vi "C8855_read_data.vi"(6 "error in (no error)":errorcluster, 7 "Cluster in":T1, 8 "Handle":i32) -> (0 "error out":errorcluster, 1 "Data update error 1":bool, 2 "Result Returned":u8, 3 "Handle 2":i32, 5 "Cluster out":T1)   [LabVIEW 2014]
uses:
  Source Cluster.ctl
  C8855-01api.dll
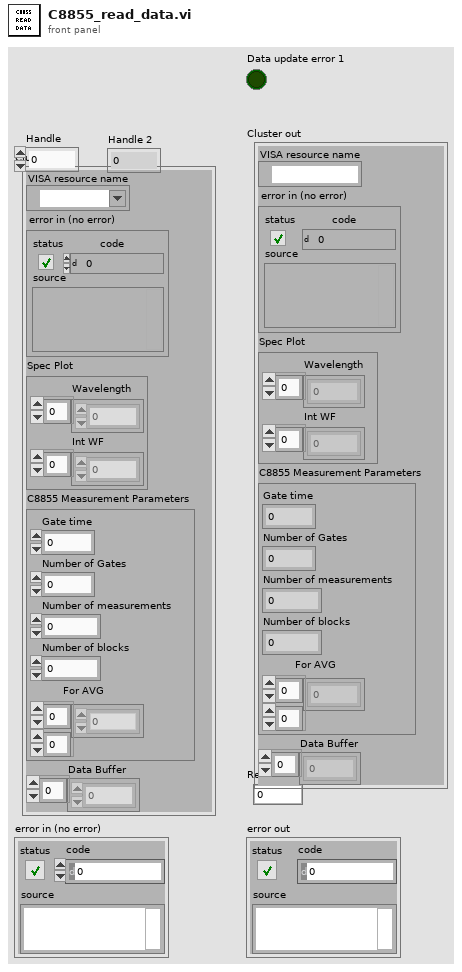
[diagram p1: front panel]
types:
  T1 = typedef "Source Cluster.ctl" = cluster{"VISA resource name":refnum<visa-resource-name>, "error in (no error)":errorcluster, "Spec Plot":cluster{"Wavelength":dbl[], "Int WF":dbl[]}, "C8855 Measurement Parameters":cluster{"Gate time":u8, "Number of Gates":u16, "Number of measurements":i32, "Number of blocks":i32, "For AVG":dbl[][]}, "Data Buffer":u32[]}
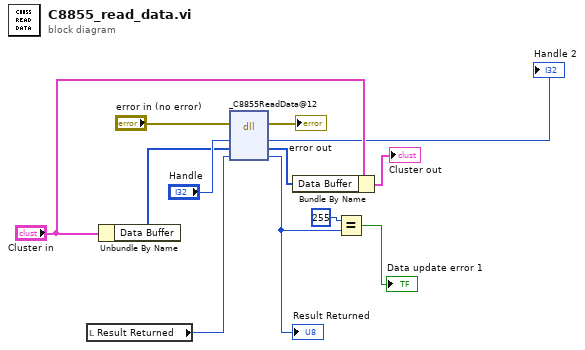
[diagram p0: block diagram]
diagram:
  n1 = local read "Result Returned"() -> (w3:u8)
  n2 = Unbundle By Name("Cluster in") -> ("Data Buffer"=w1:u32[])
  n3 = dll-call lib="C:/Users/physrin/Documents/LSLV/Labview Laser Spectroscopy/C8855-01api.dll" fn="_C8855ReadData@12"(error in="error in (no error)", "Handle"="Handle", "Data Buffer"=w1, "ResultReturned"=w3) -> (error out=→"error out":errorcluster, "Handle"=→"Handle 2":i32, "Data Buffer"=w11:u32[], "ResultReturned"=w8:u8)  [unwired: 2 in, 2 out]
  "Result Returned" <- w8
  n4 = Bundle By Name(cluster="Cluster in", "Data Buffer"=w11) -> (→"Cluster out":T1)
  n5 = Equal?(x=u8 255 ("y"), y=w8) -> (x = y?=→"Data update error 1":bool)
